vi "test_5160_stage1.vi"() -> ()   [LabVIEW 2013]
uses:
  <vilib>/measure/maspectr.llb/Power Spectrum and PSD Export Mode.ctl
  <vilib>/measure/maspectr.llb/FFT Power Spectrum and PSD for 1 Chan (CDB).vi
  <vilib>/measure/NI_MAPro.lvlib
panel:
  out "size before":i32
  out "Waveform Graph":dbl[](graph)
  out "power spectrum":cluster{"f0":dbl, "df":dbl, "magnitude":dbl[]}(graph)
  out "size after":i32
  out "Q out":fxp<+/-,16,14>[](array[numeric])
  out "I out":fxp<+/-,16,14>[](array[numeric])
  out "iteration1":i32
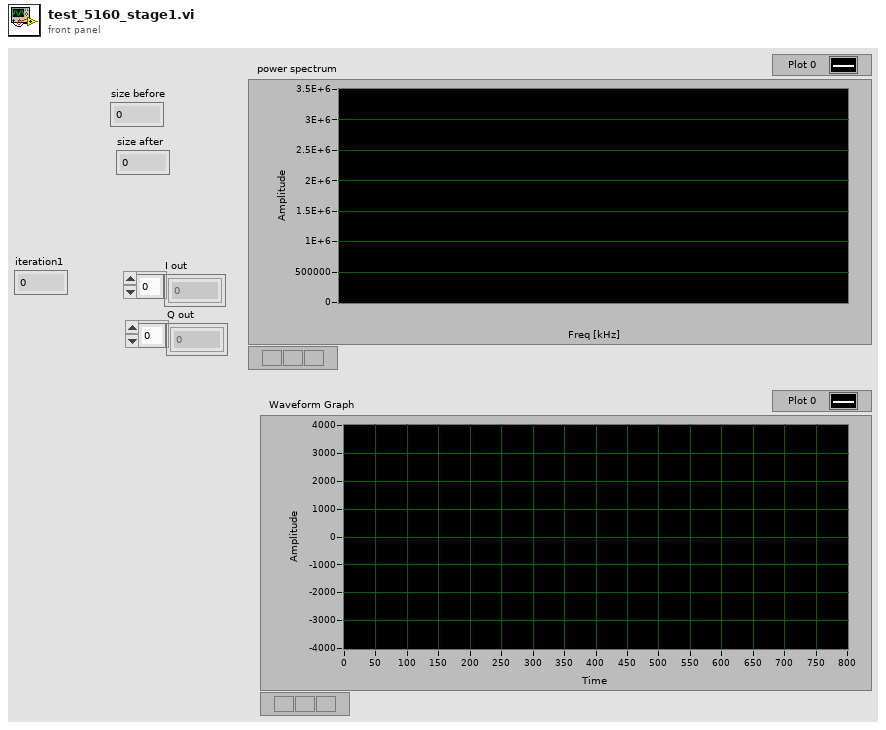
[diagram p1: front panel]
types:
  T1 = typedef "NI_MAPro.lvlib/Power Spectrum and PSD Export Mode.ctl" = u16
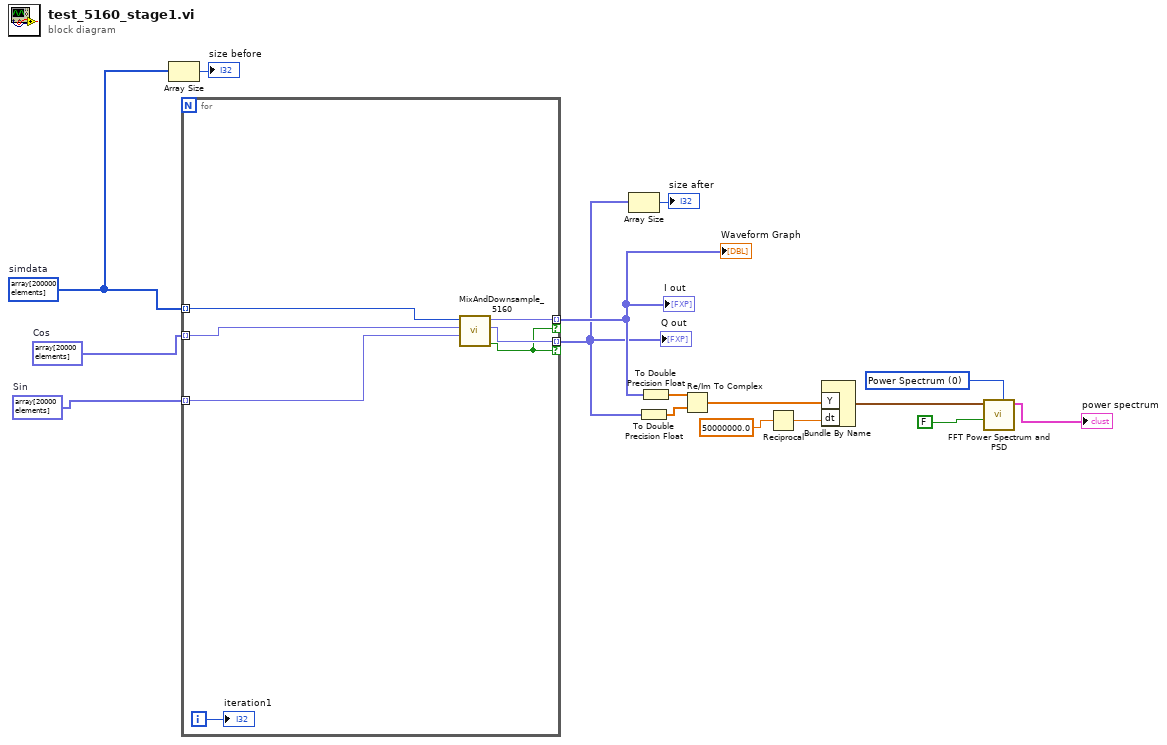
[diagram p0: block diagram]
diagram:
  w5 = fxp<+/-,16,0>[] array[20000 elements]  # Cos
  w1 = i16[] array[200000 elements]  # simdata
  w6 = fxp<+/-,16,0>[] array[20000 elements]  # Sin
  w15 = T1 0 items=["Power Spectrum", "Power Spectral Density"] ("export mode")
  n1 = Array Size(array=w1) -> (size(s)=→"size before":i32)
  n2 = for {
    tunnel: [w23] -> w4 mode=indexing if=w21
    tunnel: [w22] -> w3 mode=indexing if=w21
    tunnel: w1 -> [w19] mode=indexing
    tunnel: w5 -> [w18] mode=indexing
    tunnel: w6 -> [w17] mode=indexing
    i -> [w20]
    n3 = call "MixAndDownsample_5160.vi"("Sine in"=w17, "Cosine in"=w18, "Sample in"=w19) -> ("valid out"=w21:bool, "Q out"=w22:fxp<+/-,16,14>, "I out"=w23:fxp<+/-,16,14>)  [unwired: 6 in]
    "iteration1" <- w20
  }
  "I out" <- w4
  "Q out" <- w3
  "Waveform Graph" <- w4
  n4 = Array Size(array=w3) -> (size(s)=→"size after":i32)
  n5 = To Double Precision Float(number=w3) -> (double precision float=w8:dbl[])
  n6 = To Double Precision Float(number=w4) -> (double precision float=w9:dbl[])
  n7 = Re/Im To Complex(1:w8, 2:w9) -> (0:w7:cdb[])
  n8 = Reciprocal(x=50000000.0 ("dt")) -> (1/x=w11:dbl)
  n9 = Bundle By Name("Y"=w7, "dt"=w11) -> (w14:waveform(cdb))  [unwired: 1 in]
  n10 = call-poly <vilib>:"FFT Power Spectrum and PSD.vi"("export mode"=w15, "dB On (F)"=FALSE, "time signal"=w14) -> ("Power Spectrum / PSD"=→"power spectrum":cluster{"f0":dbl, "df":dbl, "magnitude":dbl[]})  [unwired: 5 in, 3 out]
